vi "HW3_2018.vi"() -> ()   [LabVIEW 2018]
panel:
  in  "Path":path
  in  "min":dbl
  in  "hour":dbl
  in  "OK Button":bool
  out "Boolean":bool
  in  "SET ALARM":bool
  out "ALARMING TIME":string
  out "DATE":string
  in  "reinstate":bool
  in  "sec":dbl
  in  "min":dbl
  in  "hour":dbl
  in  "reset":bool
  out "sec":dbl(knob) scale=0.0..60.0
  out "min":dbl(knob) scale=0.0..60.0
  out "hour":dbl(knob) scale=0.0..12.0
  in  "stop":bool
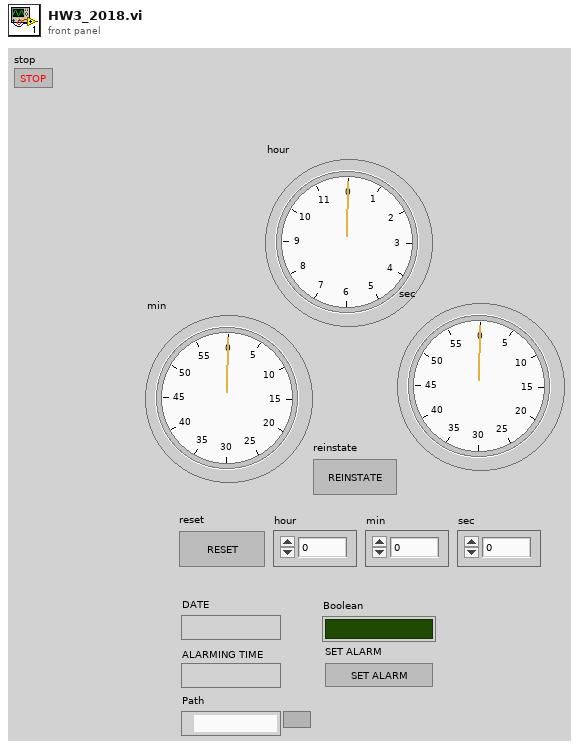
[diagram p1: front panel]
types:
  T1 = typedef "LVDateTimeRec.ctl" = cluster{"fractional second":dbl, "second":i32, "minute":i32, "hour":i32, "day of month":i32, "month":i32, "year":i32, "day of week":i32, "day of year":i32, "DST":i32}
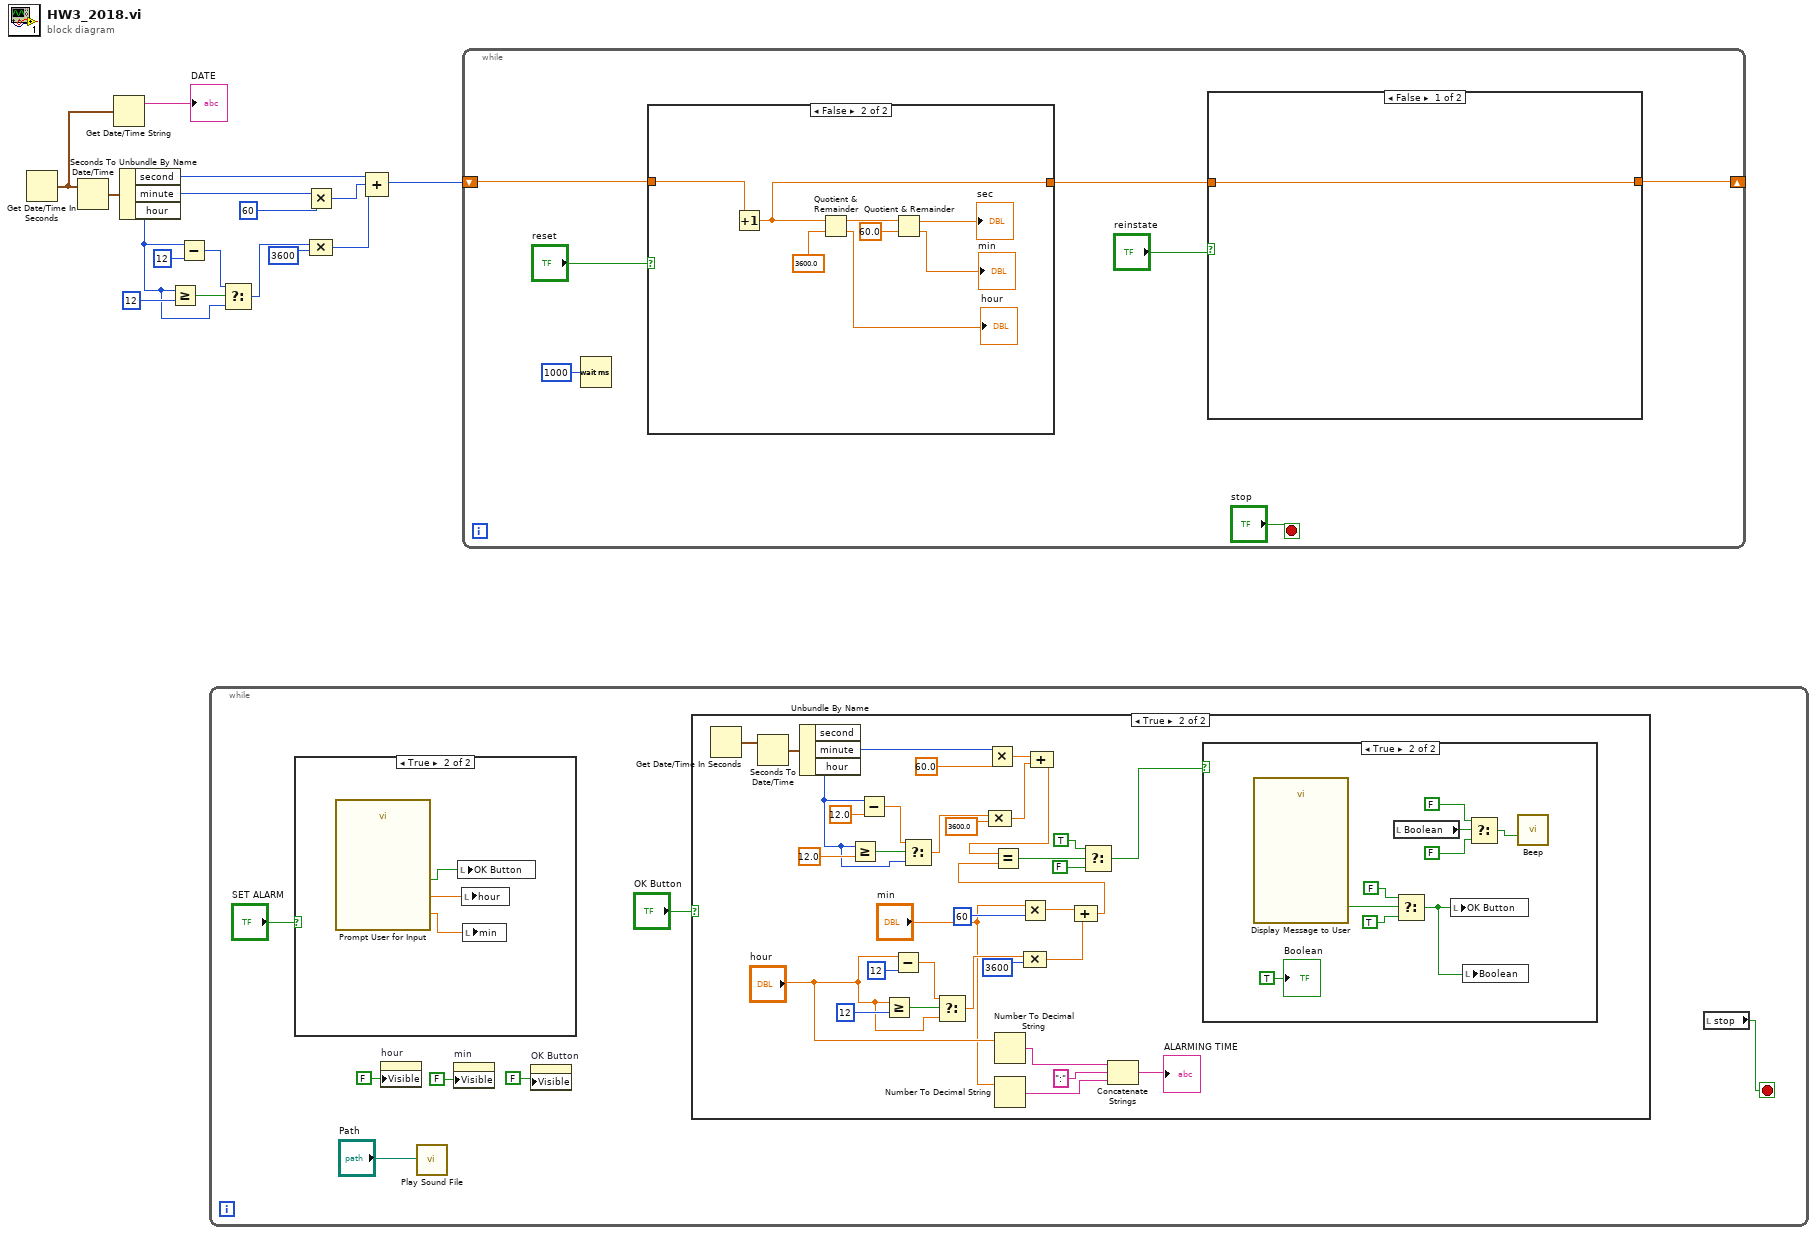
[diagram p0: block diagram]
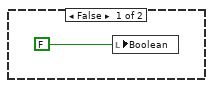
[diagram p3: hidden frame]
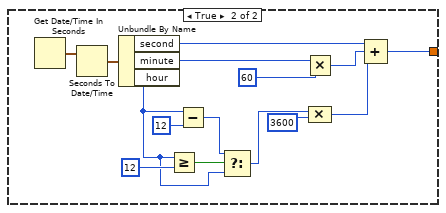
[diagram p5: hidden frame]
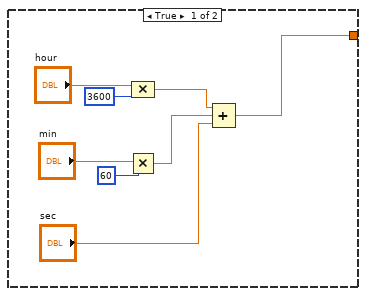
[diagram p6: hidden frame]
diagram:
  n1 = Get Date/Time In Seconds() -> (seconds since 1Jan1904=w5:timestamp)
  n2 = Seconds To Date/Time(time stamp (now)=w5) -> (date time rec=w14:T1)  [unwired: 1 in]
  n3 = Get Date/Time String(seconds (now)=w5) -> (date string=→"DATE":string)  [unwired: 2 in, 1 out]
  n4 = Unbundle By Name(w14) -> ("second"=w12:i32, "minute"=w13:i32, "hour"=w7:i32)
  n5 = Greater Or Equal?(x=w7, y=12) -> (x >= y?=w10:bool)
  n6 = Subtract(x=w7, y=12) -> (x-y=w8:i32)
  n7 = while {
    stop <- w19 stop-if-true
    n8 = case shown="True" "SET ALARM" {
      frame False {
      }
      frame True {
        n9 = call "Prompt User for Input"() -> ("Minute"=w70:dbl, "Hour"=w69:dbl, "OK"=w68:bool)  [unwired: 16 in, 1 out]
        n10 = local write "OK Button"(w68) -> ()
        n11 = local write "hour"(w69) -> ()
        n12 = local write "min"(w70) -> ()
      }
    }
    n13 = property on="hour" class="DigNum (strict)"("Visible"=FALSE) -> ()  [unwired: 2 in, 2 out]
    n14 = call <vilib>:"Play Sound File.vi"("path"="Path") -> ()  [unwired: 9 in, 2 out]
    n15 = property on="min" class="DigNum (strict)"("Visible"=FALSE) -> ()  [unwired: 2 in, 2 out]
    n16 = property on="OK Button" class="Bool (strict)"("Visible"=FALSE) -> ()  [unwired: 2 in, 2 out]
    n17 = case shown="True" "OK Button" {
      frame False {
      }
      frame True {
        n18 = Get Date/Time In Seconds() -> (seconds since 1Jan1904=w27:timestamp)
        n19 = Seconds To Date/Time(time stamp (now)=w27) -> (date time rec=w30:T1)  [unwired: 1 in]
        n20 = Unbundle By Name(w30) -> ("minute"=w31:i32, "hour"=w24:i32)  [unwired: 1 out]
        n21 = Greater Or Equal?(x=w24, y=12.0) -> (x >= y?=w33:bool)
        n22 = Subtract(x=w24, y=12.0) -> (x-y=w35:dbl)
        n23 = Greater Or Equal?(x="hour", y=12) -> (x >= y?=w52:bool)
        n24 = Subtract(x="hour", y=12) -> (x-y=w50:dbl)
        n25 = Select(t=w35, s=w33, f=w24) -> (s? t:f=w36:dbl)
        n26 = Select(t=w50, s=w52, f="hour") -> (s? t:f=w49:dbl)
        n27 = Multiply(x=w31, y=60.0) -> (x*y=w37:dbl)
        n28 = Compound Arithmetic op=MULTIPLY(w36, 3600.0) -> (w38:dbl)
        n29 = Number To Decimal String(number="hour") -> (decimal integer string=w44:string)  [unwired: 1 in]
        n30 = Number To Decimal String(number="min") -> (decimal integer string=w42:string)  [unwired: 1 in]
        n31 = Multiply(x="min", y=60) -> (x*y=w55:dbl)
        n32 = Compound Arithmetic op=MULTIPLY(w49, 3600) -> (w54:dbl)
        n33 = Compound Arithmetic op=ADD(w37, w38) -> (w26:dbl)
        n34 = Compound Arithmetic op=ADD(w55, w54) -> (w48:dbl)
        n35 = Equal?(x=w26, y=w48) -> (x = y?=w47:bool)
        n36 = Select(t=TRUE, s=w47, f=FALSE) -> (s? t:f=w25:bool)
        n37 = Concatenate Strings(w44, ":", w42) -> (→"ALARMING TIME":string)
        n38 = case shown="True" w25 {
          frame False {
            n39 = local write "Boolean"(FALSE ("Boolean")) -> ()
          }
          frame True {
            n40 = call "Display Message to User"() -> ("OK"=w66:bool)  [unwired: 10 in, 1 out]
            n41 = local read "Boolean"() -> (w62:bool)
            n42 = Select(t=FALSE ("Boolean"), s=w66, f=TRUE) -> (s? t:f=w63:bool)
            n43 = local write "OK Button"(w63) -> ()
            n44 = local write "Boolean"(w63) -> ()
            n45 = Select(t=FALSE ("Boolean"), s=w62, f=FALSE ("Boolean")) -> (s? t:f=w61:bool)
            n46 = call <vilib>:"Beep.vi"("use system alert? (T)"=w61) -> ()  [unwired: 11 in]
            "Boolean" <- TRUE ("Boolean")
          }
        }
      }
    }
    n47 = local read "stop"() -> (w19:bool)
  }
  n48 = Select(t=w8, s=w10, f=w7) -> (s? t:f=w6:i32)
  n49 = Multiply(x=w13, y=60) -> (x*y=w2:i32)
  n50 = Compound Arithmetic op=MULTIPLY(w6, 3600) -> (w1:i32)
  n51 = Compound Arithmetic op=ADD(w12, w2, w1) -> (w4:i32)
  n52 = while {
    shift-right: [w72] -> _
    shift-left: w4 -> [w76]
    stop <- "stop" stop-if-true
    n53 = Wait (ms)(milliseconds to wait=u32 1000) -> ()  [unwired: 1 out]
    n54 = case shown="False" "reset" {
      tunnel: w76 -> [_ w109]
      tunnel: [w94 w102] -> w73
      frame True {
        n55 = Multiply(x="min", y=60) -> (x*y=w96:dbl)
        n56 = Compound Arithmetic op=MULTIPLY("hour", 3600) -> (w97:dbl)
        n57 = Compound Arithmetic op=ADD(w97, w96, "sec") -> (w94:dbl)
      }
      frame False {
        n58 = Increment(x=w109) -> (x+1=w102:dbl)
        n59 = Quotient & Remainder(x=w102, y=3600.0) -> (x-y*floor(x/y)=w107:dbl, floor(x/y)=→"hour":dbl)
        n60 = Quotient & Remainder(x=w107, y=60.0) -> (x-y*floor(x/y)=→"sec":dbl, floor(x/y)=→"min":dbl)
      }
    }
    n61 = case shown="False" "reinstate" {
      tunnel: w73 -> [w78 _]
      tunnel: [w78 w79] -> w72
      frame False {
      }
      frame True {
        n62 = Get Date/Time In Seconds() -> (seconds since 1Jan1904=w90:timestamp)
        n63 = Seconds To Date/Time(time stamp (now)=w90) -> (date time rec=w89:T1)  [unwired: 1 in]
        n64 = Unbundle By Name(w89) -> ("second"=w86:i32, "minute"=w88:i32, "hour"=w81:i32)
        n65 = Greater Or Equal?(x=w81, y=12) -> (x >= y?=w84:bool)
        n66 = Subtract(x=w81, y=12) -> (x-y=w82:i32)
        n67 = Select(t=w82, s=w84, f=w81) -> (s? t:f=w80:i32)
        n68 = Multiply(x=w88, y=60) -> (x*y=w91:i32)
        n69 = Compound Arithmetic op=MULTIPLY(w80, 3600) -> (w87:i32)
        n70 = Compound Arithmetic op=ADD(w86, w91, w87) -> (w79:i32)
      }
    }
  }
